vi "test_libssh2_sftp_open_ex_r.vi"() -> ()   [LabVIEW 2017, in "integration_tests.lvlib"]
uses:
  integration_tests.lvlib
  libssh2/libssh2_sftp_attributes.ctl
  support/support.lvlib
  libssh2/libssh2.lvlib
  <vilib>/PNR/Transparent Assertions/Transparent Assertions/Transparent Assertions.lvlib
panel:
  out "error out":errorcluster
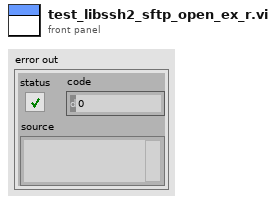
[diagram p1: front panel]
types:
  T1 = typedef "libssh2.lvlib/libssh2_sftp_attributes.ctl" = cluster{"flags":u32, "filesize":u64, "uid":u32, "gid":u32, "permissions":u32, "atime":u32, "mtime":u32}
  T2 = typedef "libssh2.lvlib/Session Refnum.ctl" = refnum<k1>
  T3 = typedef "libssh2.lvlib/SFTP Refnum.ctl" = refnum<k1>
  T4 = typedef "libssh2.lvlib/SFTP Handle Refnum.ctl" = refnum<k1>
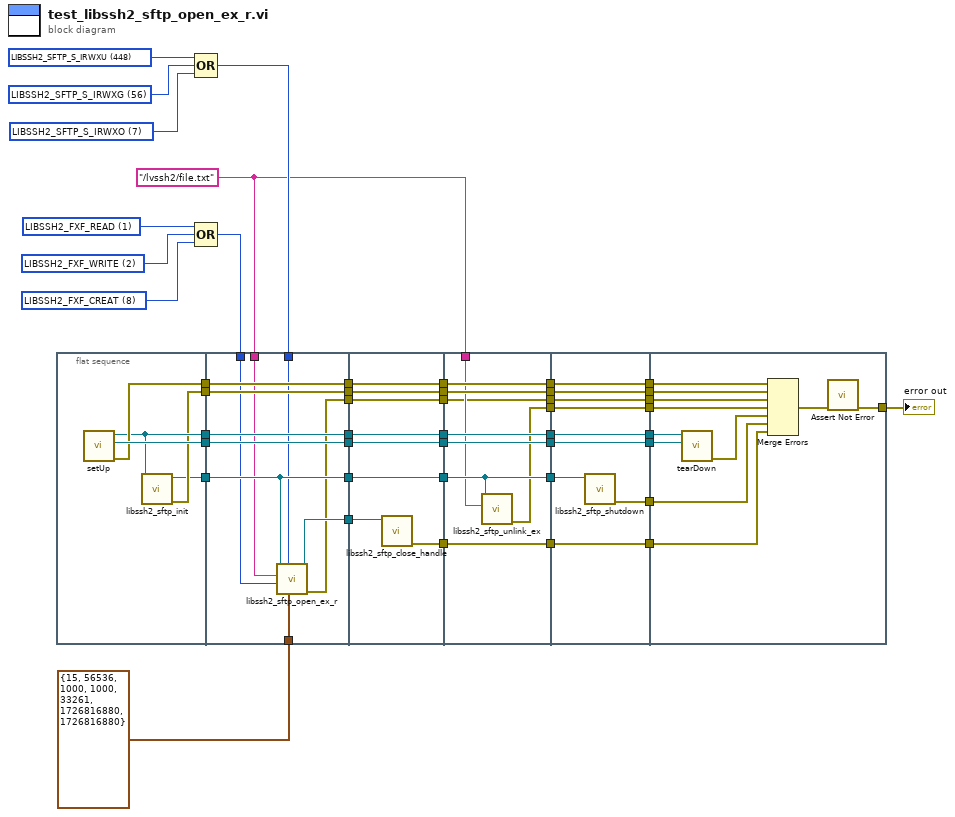
[diagram p0: block diagram]
diagram:
  w35 = u32 2 items=["LIBSSH2_FXF_READ"=1, "LIBSSH2_FXF_WRITE"=2, "LIBSSH2_FXF_APPEND"=4, "LIBSSH2_FXF_CREAT"=8, "LIBSSH2_FXF_TRUNC"=16, "LIBSSH2_FXF_EXCL"=32] ("flags")
  w36 = u32 1 items=["LIBSSH2_FXF_READ"=1, "LIBSSH2_FXF_WRITE"=2, "LIBSSH2_FXF_APPEND"=4, "LIBSSH2_FXF_CREAT"=8, "LIBSSH2_FXF_TRUNC"=16, "LIBSSH2_FXF_EXCL"=32] ("flags")
  w34 = u32 8 items=["LIBSSH2_FXF_READ"=1, "LIBSSH2_FXF_WRITE"=2, "LIBSSH2_FXF_APPEND"=4, "LIBSSH2_FXF_CREAT"=8, "LIBSSH2_FXF_TRUNC"=16, "LIBSSH2_FXF_EXCL"=32] ("flags")
  w8 = "/lvssh2/file.txt" ("filename")
  w38 = 7 items=["LIBSSH2_SFTP_S_IRWXU"=448, "LIBSSH2_SFTP_S_IRUSR"=256, "LIBSSH2_SFTP_S_IWUSR"=128, "LIBSSH2_SFTP_S_IXUSR"=64, "LIBSSH2_SFTP_S_IRWXG"=56, "LIBSSH2_SFTP_S_IRGRP"=32, "LIBSSH2_SFTP_S_IWGRP"=16, "LIBSSH2_SFTP_S_IXGRP"=8, "LIBSSH2_SFTP_S_IRWXO"=7, "LIBSSH2_SFTP_S_IROTH"=4, "LIBSSH2_SFTP_S_IWOTH"=2, "LIBSSH2_SFTP_S_IXOTH"=1] ("mode")
  w39 = 56 items=["LIBSSH2_SFTP_S_IRWXU"=448, "LIBSSH2_SFTP_S_IRUSR"=256, "LIBSSH2_SFTP_S_IWUSR"=128, "LIBSSH2_SFTP_S_IXUSR"=64, "LIBSSH2_SFTP_S_IRWXG"=56, "LIBSSH2_SFTP_S_IRGRP"=32, "LIBSSH2_SFTP_S_IWGRP"=16, "LIBSSH2_SFTP_S_IXGRP"=8, "LIBSSH2_SFTP_S_IRWXO"=7, "LIBSSH2_SFTP_S_IROTH"=4, "LIBSSH2_SFTP_S_IWOTH"=2, "LIBSSH2_SFTP_S_IXOTH"=1] ("mode")
  w40 = 448 items=["LIBSSH2_SFTP_S_IRWXU"=448, "LIBSSH2_SFTP_S_IRUSR"=256, "LIBSSH2_SFTP_S_IWUSR"=128, "LIBSSH2_SFTP_S_IXUSR"=64, "LIBSSH2_SFTP_S_IRWXG"=56, "LIBSSH2_SFTP_S_IRGRP"=32, "LIBSSH2_SFTP_S_IWGRP"=16, "LIBSSH2_SFTP_S_IXGRP"=8, "LIBSSH2_SFTP_S_IRWXO"=7, "LIBSSH2_SFTP_S_IROTH"=4, "LIBSSH2_SFTP_S_IWOTH"=2, "LIBSSH2_SFTP_S_IXOTH"=1] ("mode")
  n1 = flat-sequence {
    tunnel: [w49] -> w46
    tunnel: [w51] -> w45
    tunnel: [w50] -> w44
    tunnel: [w48] -> w42
    tunnel: [w47] -> w41
    tunnel: w46 -> [w62]
    tunnel: w45 -> [w61]
    tunnel: [w62] -> w26
    tunnel: [w61] -> w25
    tunnel: [w58] -> w24
    tunnel: [w60] -> w23
    tunnel: w44 -> [w60]
    tunnel: w42 -> [w59]
    tunnel: [w59] -> w22
    tunnel: w41 -> [w58]
    tunnel: w37 -> [w57]
    tunnel: w8 -> [w56]
    tunnel: w33 -> [w55]
    tunnel: [w54] -> w21
    tunnel: T1 {"flags"=15, "filesize"=56536, "uid"=1000, "gid"=1000, "permissions"=33261, "atime"=1726816880, "mtime"=1726816880} ("attributes") -> [w53]
    tunnel: [w52] -> w4
    tunnel: w26 -> [w70]
    tunnel: [w70] -> w20
    tunnel: w25 -> [w69]
    tunnel: [w69] -> w18
    tunnel: w24 -> [w68]
    tunnel: [w68] -> w16
    tunnel: w23 -> [w67]
    tunnel: [w67] -> w14
    tunnel: w22 -> [w66]
    tunnel: [w66] -> w12
    tunnel: w21 -> [w65]
    tunnel: [w64] -> w10
    tunnel: w4 -> [w63]
    tunnel: [w63] -> w3
    tunnel: w20 -> [w79]
    tunnel: [w79] -> w19
    tunnel: w18 -> [w78]
    tunnel: [w78] -> w17
    tunnel: w16 -> [w74]
    tunnel: [w74] -> w15
    tunnel: w14 -> [w77]
    tunnel: [w77] -> w13
    tunnel: w12 -> [w76]
    tunnel: [w76] -> w11
    tunnel: w10 -> [w75]
    tunnel: [w75] -> w9
    tunnel: w8 -> [w73]
    tunnel: [w72] -> w7
    tunnel: w3 -> [w71]
    tunnel: [w71] -> w2
    tunnel: w19 -> [w88]
    tunnel: [w88] -> w32
    tunnel: w17 -> [w87]
    tunnel: [w87] -> w31
    tunnel: w15 -> [w84]
    tunnel: w13 -> [w86]
    tunnel: [w86] -> w30
    tunnel: w11 -> [w85]
    tunnel: [w85] -> w29
    tunnel: [w83] -> w28
    tunnel: [w82] -> w27
    tunnel: w9 -> [w82]
    tunnel: w7 -> [w81]
    tunnel: [w81] -> w6
    tunnel: w2 -> [w80]
    tunnel: [w80] -> w1
    tunnel: w32 -> [w99]
    tunnel: w31 -> [w98]
    tunnel: w30 -> [w97]
    tunnel: [w94] -> w43
    tunnel: w29 -> [w93]
    tunnel: w28 -> [w92]
    tunnel: w27 -> [w91]
    tunnel: w6 -> [w90]
    tunnel: w1 -> [w89]
    frame #0 {
      n2 = call "setUp.vi"() -> ("error out"=w50:errorcluster, "connection ID"=w51:refnum<k5>, "session"=w49:T2)  [unwired: 9 in]
      n3 = call "libssh2_sftp_init.vi"("session"=w49) -> ("error out"=w48:errorcluster, "sftp"=w47:T3)  [unwired: 9 in]
    }
    frame #1 {
      n4 = call "libssh2_sftp_open_ex_r.vi"("attributes"=w53, "mode"=w57, "flags"=w55, "filename"=w56, "sftp"=w58) -> ("error out"=w52:errorcluster, "sftp handle"=w54:T4)  [unwired: 5 in]
    }
    frame #2 {
      n5 = call "libssh2_sftp_close_handle.vi"("sftp handle"=w65) -> ("error out"=w64:errorcluster)  [unwired: 10 in]
    }
    frame #3 {
      n6 = call "libssh2_sftp_unlink_ex.vi"("file"=w73, "sftp"=w74) -> ("error out"=w72:errorcluster)  [unwired: 9 in]
    }
    frame #4 {
      n7 = call "libssh2_sftp_shutdown.vi"("sftp"=w84) -> ("error out"=w83:errorcluster)  [unwired: 10 in]
    }
    frame #5 {
      n8 = call "tearDown.vi"("connection ID"=w98, "session"=w99) -> ("error out"=w96:errorcluster)  [unwired: 9 in]
      n9 = Merge Errors(w97, w93, w89, w90, w96, w92, w91) -> (w95:errorcluster)
      n10 = call <vilib>:"Assert Not Error.vi"("error in (no error)"=w95) -> ("error out"=w94:errorcluster)  [unwired: 10 in]
    }
  }
  n11 = Compound Arithmetic op=OR(w40, w39, w38) -> (w37:i32)
  n12 = Compound Arithmetic op=OR(w36, w35, w34) -> (w33:u32)
  "error out" <- w43
